vi "Reset.vi"(8 "error in (no error)":errorcluster, 11 "MSOX6004 in":refnum<class "MSOX6004.lvclass">) -> (0 "error out":errorcluster, 3 "MSOX6004 out":refnum<class "MSOX6004.lvclass">)   [LabVIEW 2018, in "MSOX6004.lvlib" / "MSOX6004.lvclass"]
uses:
  MSOX6004.lvclass
  MSOX6004.lvclass/MSOX6004.ctl
  <instrlib>/Keysight InfiniiVision/Keysight InfiniiVision.lvlib
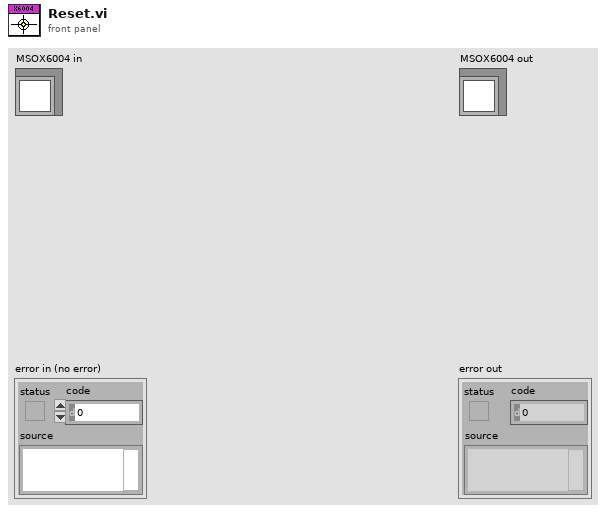
[diagram p1: front panel]
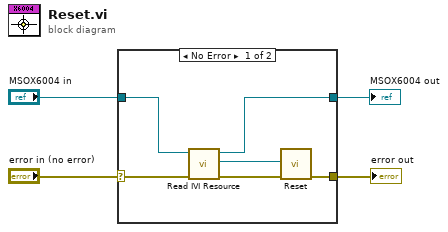
[diagram p0: block diagram]
diagram:
  n1 = case shown="No Error" "error in (no error)" {
    selector: "error in (no error)" -> [w10 w11]
    tunnel: "MSOX6004 in" -> [w9 w12]
    tunnel: [w6 w12] -> w2
    tunnel: [w5 w11] -> w1
    frame No Error {
      n2 = call "Read IVI Resource.vi"("error in (no error)"=w10, "MSOX6004 in"=w9) -> ("error out"=w7:errorcluster, "IVI Resource"=w8:refnum<k15>, "MSOX6004 out"=w6:refnum<class "MSOX6004.lvclass">)  [unwired: 7 in]
      n3 = call <instrlib>:"Reset.vi"("error in (no error)"=w7, "instrument handle"=w8) -> ("error out"=w5:errorcluster)  [unwired: 8 in, 1 out]
    }
    frame Error {
    }
  }
  "error out" <- w1
  "MSOX6004 out" <- w2
